vi "OutBitsCheckSingleCmd.vi"() -> ()   [LabVIEW 2014]
panel:
  in  "actStep":i32
  in  "stepChanged":bool
  in  "scanChanged":bool
  in  "actScan":i32
  out "outbit_out":bool
  in  "outbit_in":bool
  in  "CMDin":u32
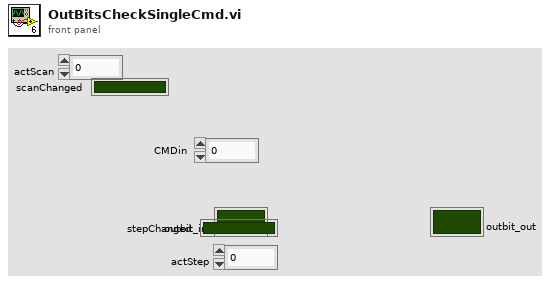
[diagram p1: front panel]
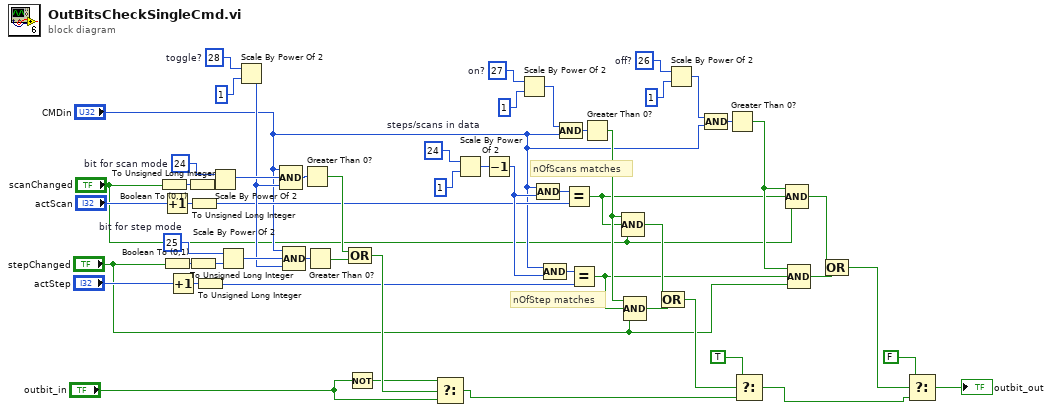
[diagram p0: block diagram]
diagram:
  w45 = i16 24  # steps/scans in data
  w47 = i16 26  # off?
  w49 = i16 27  # on?
  w51 = i16 28  # toggle?
  w54 = i16 24  # bit for scan mode
  w56 = i16 25  # bit for step mode
  # "nOfScans matches"
  # "nOfStep matches"
  n1 = Boolean To (0,1)(Boolean="scanChanged") -> (0, 1=w53:i16)
  n2 = Increment(x="actScan") -> (x+1=w31:i32)
  n3 = Boolean To (0,1)(Boolean="stepChanged") -> (0, 1=w55:i16)
  n4 = Increment(x="actStep") -> (x+1=w30:i32)
  n5 = To Unsigned Long Integer(number=w53) -> (unsigned 32bit integer=w42:u32)
  n6 = To Unsigned Long Integer(number=w55) -> (unsigned 32bit integer=w41:u32)
  n7 = To Unsigned Long Integer(number=w31) -> (unsigned 32bit integer=w24:u32)
  n8 = To Unsigned Long Integer(number=w30) -> (unsigned 32bit integer=w22:u32)
  n9 = Scale By Power Of 2(n=w54, x=w42) -> (x*2^n=w43:u32)
  n10 = Scale By Power Of 2(n=w56, x=w41) -> (x*2^n=w39:u32)
  n11 = Scale By Power Of 2(n=w51, x=u32 1 ("Data")) -> (x*2^n=w27:u32)
  n12 = Compound Arithmetic op=AND("CMDin", w43, w27) -> (w52:u32)
  n13 = Compound Arithmetic op=AND("CMDin", w39, w27) -> (w40:u32)
  n14 = Greater Than 0?(x=w52) -> (x > 0?=w26:bool)
  n15 = Greater Than 0?(x=w40) -> (x > 0?=w25:bool)
  n16 = Not(x="outbit_in") -> (.not. x?=w36:bool)
  n17 = Compound Arithmetic op=OR(w26, w25) -> (w38:bool)
  n18 = Select(t=w36, s=w38, f="outbit_in") -> (s? t:f=w17:bool)
  n19 = Scale By Power Of 2(n=w45, x=u32 1 ("Data")) -> (x*2^n=w33:u32)
  n20 = Decrement(x=w33) -> (x-1=w28:u32)
  n21 = Scale By Power Of 2(n=w49, x=u32 1 ("Data")) -> (x*2^n=w34:u32)
  n22 = Compound Arithmetic op=AND("CMDin", w28) -> (w23:u32)
  n23 = Compound Arithmetic op=AND("CMDin", w28) -> (w21:u32)
  n24 = Compound Arithmetic op=AND(w34, "CMDin") -> (w35:u32)
  n25 = Equal?(x=w23, y=w24) -> (x = y?=w8:bool)
  n26 = Equal?(x=w21, y=w22) -> (x = y?=w7:bool)
  n27 = Greater Than 0?(x=w35) -> (x > 0?=w20:bool)
  n28 = Compound Arithmetic op=AND(w20, w8, "scanChanged") -> (w18:bool)
  n29 = Compound Arithmetic op=AND(w20, w7, "stepChanged") -> (w19:bool)
  n30 = Compound Arithmetic op=OR(w18, w19) -> (w16:bool)
  n31 = Scale By Power Of 2(n=w47, x=u32 1 ("Data")) -> (x*2^n=w12:u32)
  n32 = Compound Arithmetic op=AND(w12, "CMDin") -> (w14:u32)
  n33 = Greater Than 0?(x=w14) -> (x > 0?=w9:bool)
  n34 = Select(t=TRUE, s=w16, f=w17) -> (s? t:f=w2:bool)
  n35 = Compound Arithmetic op=AND(w9, w8, "scanChanged") -> (w10:bool)
  n36 = Compound Arithmetic op=AND(w9, w7, "stepChanged") -> (w11:bool)
  n37 = Compound Arithmetic op=OR(w10, w11) -> (w3:bool)
  n38 = Select(t=FALSE, s=w3, f=w2) -> (s? t:f=→"outbit_out":bool)
